vi "XML_GetTag.vi"(11 "XML":T1) -> (0 "TAG":string, 3 "XML(dup)":T1)   [LabVIEW 2017]
doc: "Returns the name of the outermost tag in XML."
uses:
  _XML--String.ctl
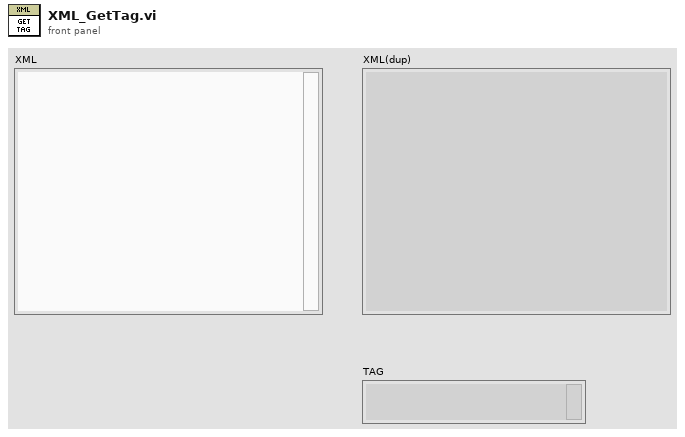
[diagram p1: front panel]
types:
  T1 = typedef "_XML--String.ctl" = string
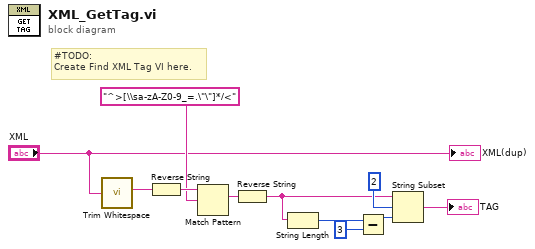
[diagram p0: block diagram]
diagram:
  # "#TODO:\nCreate Find XML Tag VI here."
  n1 = call <vilib>:"Trim Whitespace.vi"("string"="XML") -> ("trimmed string"=w9:string)  [unwired: 1 in]
  n2 = Reverse String(1:w9) -> (0:w11:string)
  n3 = Match Pattern(string=w11, regular expression="^>[\\sa-zA-Z0-9_=.\"\"]*/<" ("string")) -> (match substring=w8:string)  [unwired: 1 in, 3 out]
  n4 = Reverse String(1:w8) -> (0:w6:string)
  n5 = String Length(string=w6) -> (length=w5:i32)
  n6 = Subtract(x=w5, y=3) -> (x-y=w4:i32)
  n7 = String Subset(string=w6, offset (0)=2, length (rest)=w4) -> (substring=→"TAG":string)
  "XML(dup)" <- "XML"
